vi "Resistance to temperature.vi"(9 "B":dbl=3950.0, 10 "Resistance":dbl, 11 "R0":dbl=10000.0) -> (3 "Temperature":dbl)   [LabVIEW 2022 SP3]
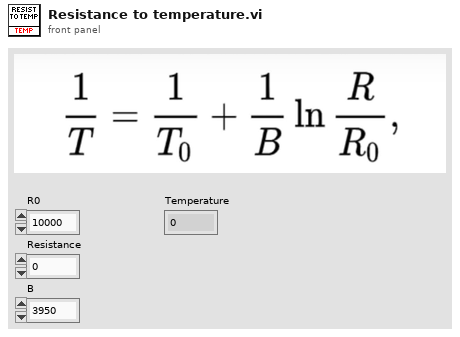
[diagram p1: front panel]
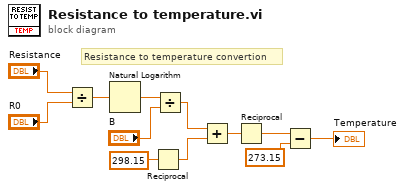
[diagram p0: block diagram]
diagram:
  # "Resistance to temperature convertion"
  n1 = Divide(x="Resistance", y="R0") -> (x/y=w10:dbl)
  n2 = Natural Logarithm(1:w10) -> (0:w4:dbl)
  n3 = Reciprocal(x=298.15) -> (1/x=w7:dbl)
  n4 = Divide(x=w4, y="B") -> (x/y=w8:dbl)
  n5 = Add(x=w8, y=w7) -> (x+y=w6:dbl)
  n6 = Reciprocal(x=w6) -> (1/x=w3:dbl)
  n7 = Subtract(x=w3, y=273.15) -> (x-y=→"Temperature":dbl)
